vi "Set velocity.vi"(8 "error in (no error)":errorcluster, 10 "Velocity (rev/sec)":dbl, 11 "AlphaStep One in":refnum<class "AlphaStep One.lvclass">) -> (0 "error out":errorcluster, 3 "AlphaStep One out":refnum<class "AlphaStep One.lvclass">)   [LabVIEW 2015, in "AlphaStep One.lvclass"]
uses:
  AlphaStep One.lvclass
  AlphaStep One.lvclass/AlphaStep One.ctl
  Serial Device/Serial Device.lvclass
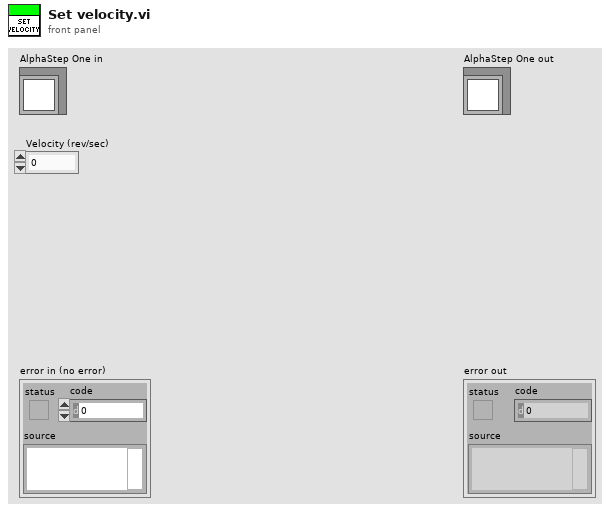
[diagram p1: front panel]
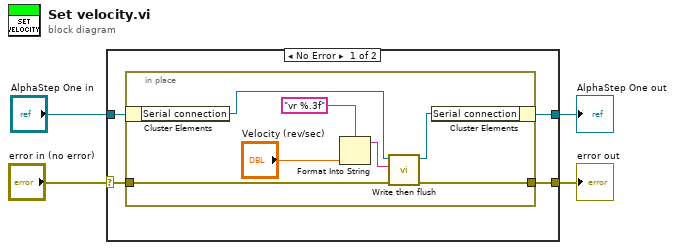
[diagram p0: block diagram]
diagram:
  n1 = case shown="No Error" "error in (no error)" {
    selector: "error in (no error)" -> [w7 w17]
    tunnel: [w6 w17] -> w3
    tunnel: "AlphaStep One in" -> [w8 w16]
    tunnel: [w5 w16] -> w1
    frame No Error {
      n2 = in-place {
        in-place-border: w7 -> [w10]
        in-place-border: [w9] -> w6
        n3 = in-place-cluster #1(w8) -> ("Serial connection"=w15:refnum<class "Serial Device.lvclass">)
        n4 = Format Into String(format string="vr %.3f", "Velocity (rev/sec)") -> (resulting string=w12:string)  [unwired: 2 in, 1 out]
        n5 = call "Write then flush.vi"("error in (no error)"=w10, "TX Data"=w12, "Serial Device in"=w15) -> ("error out"=w9:errorcluster, "Serial Device out"=w11:refnum<class "Serial Device.lvclass">)  [unwired: 7 in]
        n6 = in-place-cluster #1("Serial connection"=w11) -> (w5:refnum<class "AlphaStep One.lvclass">)
      }
    }
    frame Error {
    }
  }
  "error out" <- w3
  "AlphaStep One out" <- w1
